vi "Exclude_OK.vi"(0 "Probe Volume":cluster{"Max":dbl, "Min":dbl}[](array[cluster]) {"Min" format="%.2f"; "Max" format="%.2f"}, 1 "Traverse Name":string, 2 "Previous Probe Volume":cluster{"Max":dbl, "Min":dbl}[](array[cluster]) {"Min" format="%.2f"; "Max" format="%.2f"}, 3 "Exclude Array":T1[](array[typedef]) {"Sizes"."Min" format="%#.1f"; "Sizes"."Max" format="%#.1f"}, 4 "Volume Name":string) -> (5 "Probe OK?":bool, 6 "Separation Distance":dbl format="%.2f", 7 "Error Comments":string)   [LabVIEW 2013]
uses:
  Exclude_cluster.ctl
  Box_size.ctl
  Exclusion_type.ctl
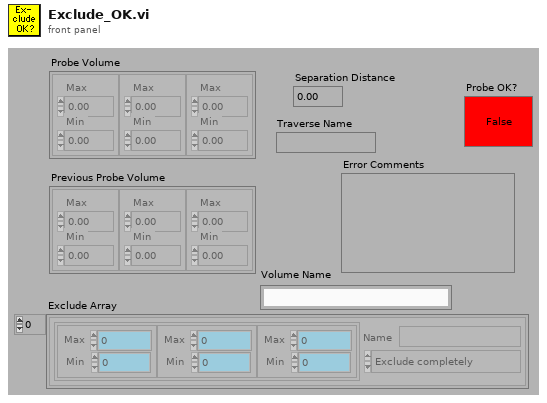
[diagram p1: front panel]
types:
  T1 = typedef "Exclude_cluster.ctl" = cluster{"Sizes":T2, "Name":string, "Exclude Type":T3}
  T2 = typedef "Box_size.ctl" = cluster{"Max":dbl, "Min":dbl}[]
  T3 = typedef "Exclusion_type.ctl" = enum16{"Exclude completely", "Allow only vertical moves"}
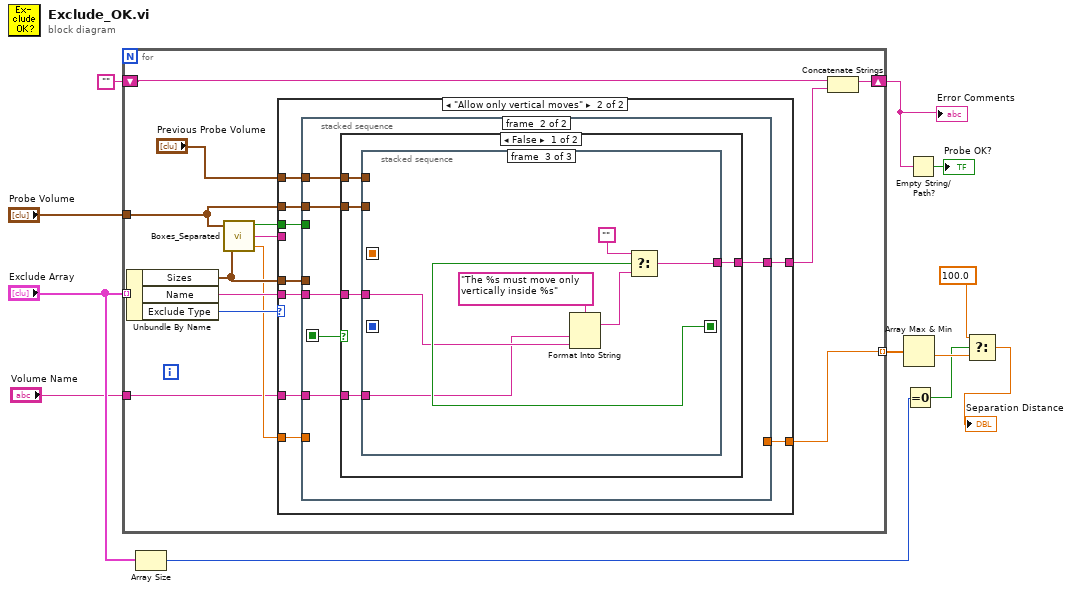
[diagram p0: block diagram]
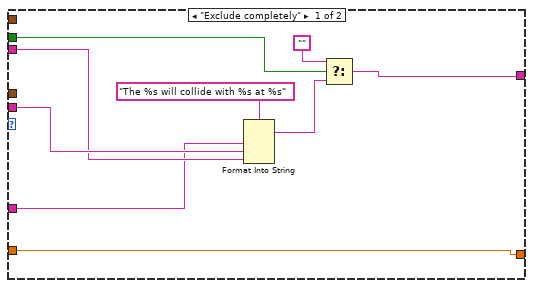
[diagram p2: hidden frame]
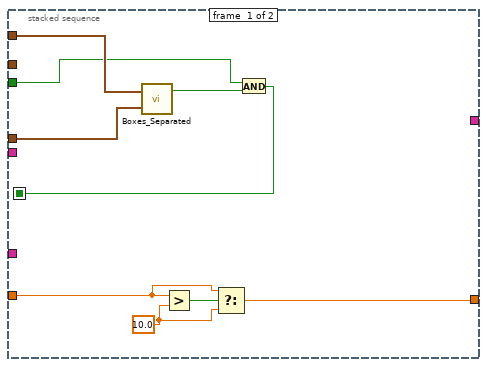
[diagram p3: hidden frame]
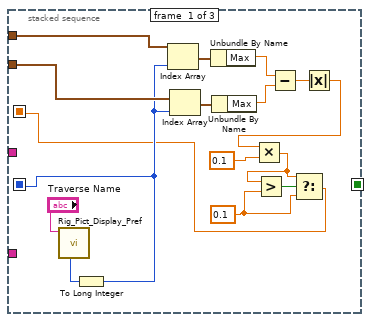
[diagram p4: hidden frame]
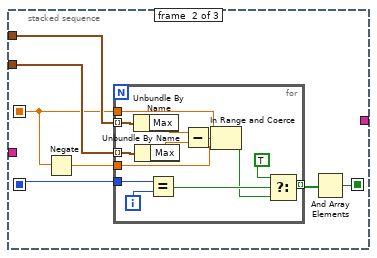
[diagram p5: hidden frame]
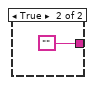
[diagram p6: hidden frame]
diagram:
  n1 = for {
    tunnel: "Exclude Array" -> [w26] mode=indexing
    tunnel: "Probe Volume" -> [w19]
    shift-right: [w20] -> w10
    shift-left: "" -> [w22]
    tunnel: [w14] -> w8 mode=indexing
    tunnel: "Volume Name" -> [w13]
    n2 = Unbundle By Name(w26) -> ("Sizes"=w17:T2, "Name"=w24:string, "Exclude Type"=w25:T3)
    n3 = call "Boxes_Separated.vi"("Box 1"=w19, "Box 2"=w17) -> ("Box Separated"=w23:bool, "Error String"=w16:string, "Separation Distance"=w15:dbl)
    n4 = case shown="\"Allow only vertical moves\"" w25 {
      tunnel: w24 -> [w34 w41]
      tunnel: w23 -> [w33 w44]
      tunnel: [w30 w43] -> w21
      tunnel: w19 -> [_ w42]
      tunnel: "Previous Probe Volume" -> [_ w40]
      tunnel: w17 -> [_ w39]
      tunnel: w16 -> [w29 _]
      tunnel: w15 -> [w28 w38]
      tunnel: [w28 w37] -> w14
      tunnel: w13 -> [w27 w36]
      frame "Exclude completely" {
        n5 = Format Into String(format string="The %s will collide with %s at %s" ("Format String"), w27, w34, w29) -> (resulting string=w32:string)  [unwired: 2 in, 1 out]
        n6 = Select(t="", s=w33, f=w32) -> (s? t:f=w30:string)
      }
      frame "Allow only vertical moves" {
        n7 = stacked-sequence {
          seq-local: [w49 _] -> [_ w55]
          tunnel: w44 -> [w50 _]
          tunnel: [_ w59] -> w43
          tunnel: w42 -> [_ w58]
          tunnel: w41 -> [_ w57]
          tunnel: w40 -> [w53 w56]
          tunnel: w39 -> [w52 _]
          tunnel: w38 -> [w47 _]
          tunnel: [w45 _] -> w37
          tunnel: w36 -> [_ w54]
          frame #0 {
            w46 = 10.0 ("y")
            n8 = call "Boxes_Separated.vi"("Box 1"=w53, "Box 2"=w52) -> ("Box Separated"=w51:bool)  [unwired: 2 out]
            n9 = Greater?(x=w47, y=w46) -> (0:w48:bool)
            n10 = Select(t=w47, s=w48, f=w46) -> (s? t:f=w45:dbl)
            n11 = And(x=w50, y=w51) -> (x .and. y?=w49:bool)
          }
          frame #1 {
            n12 = case shown="False" w55 {
              tunnel: [w62 ""] -> w59
              tunnel: w58 -> [w64 _]
              tunnel: w57 -> [w63 _]
              tunnel: w56 -> [w61 _]
              tunnel: w54 -> [w60 _]
              frame False {
                n13 = stacked-sequence {
                  seq-local: [_ w85 _] -> [_ _ w104]
                  seq-local: [w76 _ _] -> [_ w83 _]
                  seq-local: [w65 _ _] -> [_ w82 _]
                  tunnel: w64 -> [w77 w87 _]
                  tunnel: w63 -> [_ _ w103]
                  tunnel: [_ _ w102] -> w62
                  tunnel: w61 -> [w78 w84 _]
                  tunnel: w60 -> [_ _ w101]
                  frame #0 {
                    w66 = 0.1 ("y")
                    n14 = call "Rig_Pict_Display_Pref.vi"("Traverse Name"="Traverse Name") -> ("Which Axis is vertical?"=w80:enum16{"X Axis", "Y Axis", "Z Axis"})  [unwired: 7 out]
                    n15 = To Long Integer(number=w80) -> (32bit integer=w76:i32)
                    n16 = Index Array(array=w78, index=w76) -> (element=w75:cluster{"Max":dbl, "Min":dbl})
                    n17 = Index Array(array=w77, index=w76) -> (element=w74:cluster{"Max":dbl, "Min":dbl})
                    n18 = Unbundle By Name(w75) -> ("Max"=w73:dbl)
                    n19 = Unbundle By Name(w74) -> ("Max"=w72:dbl)
                    n20 = Subtract(x=w73, y=w72) -> (x-y=w71:dbl)
                    n21 = Absolute Value(x=w71) -> (abs(x)=w70:dbl)
                    n22 = Multiply(x=w70, y=0.1) -> (x*y=w67:dbl)
                    n23 = Greater?(x=w67, y=w66) -> (0:w68:bool)
                    n24 = Select(t=w67, s=w68, f=w66) -> (s? t:f=w65:dbl)
                  }
                  frame #1 {
                    n25 = Negate(x=w82) -> (-x=w81:dbl)
                    n26 = for {
                      tunnel: w84 -> [w100] mode=indexing
                      tunnel: w87 -> [w99] mode=indexing
                      tunnel: w83 -> [w98]
                      tunnel: [w94] -> w86 mode=indexing
                      tunnel: w82 -> [w89]
                      tunnel: w81 -> [w88]
                      i -> [w97]
                      n27 = Unbundle By Name(w100) -> ("Max"=w93:dbl)
                      n28 = Unbundle By Name(w99) -> ("Max"=w92:dbl)
                      n29 = Equal?(x=w98, y=w97) -> (x = y?=w96:bool)
                      n30 = Subtract(x=w93, y=w92) -> (x-y=w91:dbl)
                      n31 = In Range and Coerce(upper limit=w89, x=w91, lower limit=w88) -> (In Range?=w90:bool)  [unwired: 1 out]
                      n32 = Select(t=TRUE, s=w96, f=w90) -> (s? t:f=w94:bool)
                    }
                    n33 = And Array Elements(Boolean array=w86) -> (logical AND=w85:bool)
                  }
                  frame #2 {
                    n34 = Format Into String(format string="The %s must move only vertically inside %s" ("Format String"), w101, w103) -> (resulting string=w106:string)  [unwired: 2 in, 1 out]
                    n35 = Select(t="", s=w104, f=w106) -> (s? t:f=w102:string)
                  }
                }
              }
              frame True {
              }
            }
          }
        }
      }
    }
    n36 = Concatenate Strings(w22, w21) -> (w20:string)
  }
  "Error Comments" <- w10
  n37 = Array Size(array="Exclude Array") -> (size(s)=w2:i32)
  n38 = Array Max & Min(array=w8) -> (min value=w7:dbl)  [unwired: 3 out]
  n39 = Equal To 0?(x=w2) -> (x = 0?=w6:bool)
  n40 = Empty String/Path?(string/path=w10) -> (empty?=→"Probe OK?":bool)
  n41 = Select(t=100.0, s=w6, f=w7) -> (s? t:f=→"Separation Distance":dbl)
